vi "Send Command.vi"(8 "error in (no error)":errorcluster, 10 "Command":string) -> (0 "error out":errorcluster)   [LabVIEW 2016]
uses:
  Variables/MyRIO Lidar Class Data.vi
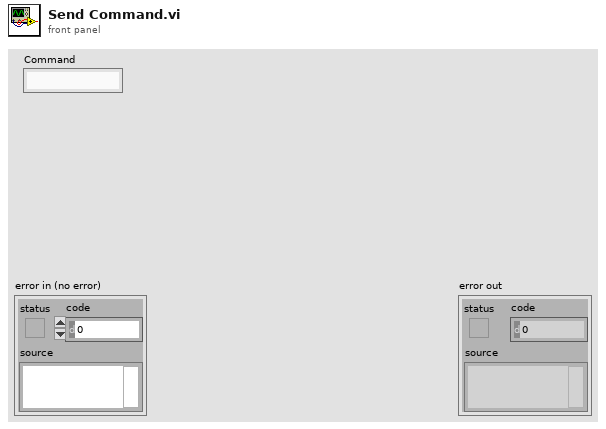
[diagram p1: front panel]
types:
  T1 = cluster{"Shared library path":path, "File Descriptor":i32}
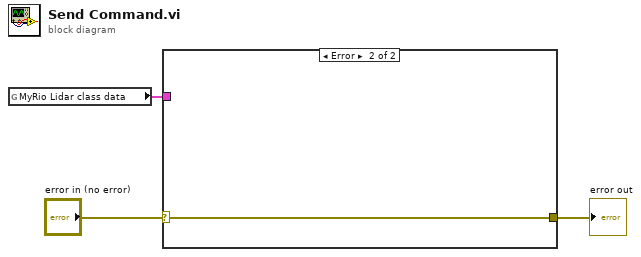
[diagram p0: block diagram]
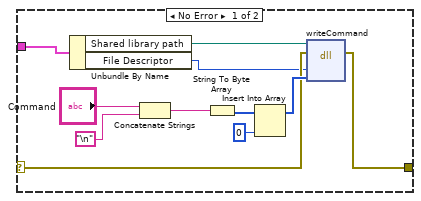
[diagram p2: hidden frame]
diagram:
  n1 = global read "MyRIO Lidar Class Data.vi" "MyRio Lidar class data"() -> (w1:T1)
  n2 = case shown="Error" "error in (no error)" {
    selector: "error in (no error)" -> [w8 w15]
    tunnel: [w7 w15] -> w2
    tunnel: w1 -> [w4 _]
    frame No Error {
      n3 = Unbundle By Name(w4) -> ("Shared library path"=w6:path, "File Descriptor"=w5:i32)
      n4 = Concatenate Strings("Command", "\n") -> (w11:string)
      n5 = String To Byte Array(string=w11) -> (unsigned byte array=w14:u8[])
      n6 = Insert Into Array(array=w14, new element=u8 0 ("new element/subarray")) -> (w12:u8[])  [unwired: 1 in]
      n7 = dll-call lib="?" fn="writeCommand"(path in=w6, error in=w8, "fd"=w5, "command"=w12) -> (error out=w7:errorcluster)  [unwired: 4 in, 1 out]
    }
    frame Error {
    }
  }
  "error out" <- w2
